vi "Angle.vi"() -> ()   [LabVIEW 2013]
panel:
  in  "Angular Data":dbl[](array[numeric])
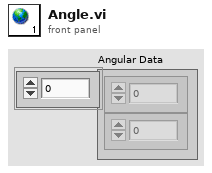
[diagram p1: front panel]
diagram:
